vi "LVFinal.vi"() -> ()   [LabVIEW 2016]
panel:
  out "Ball Color":string[](array[string])
  out "Ball Y":dbl[](array[numeric])
  out "Ball X":dbl[](array[numeric])
  in  "Send Button":bool
  in  "DAC2":dbl
  in  "DAC1":dbl
  out "Angle":dbl
  out "Velocity":dbl
  out "Y":dbl
  out "X":dbl
  in  "stop":bool
  in  "Display History":bool
  out "2D Picture":picture
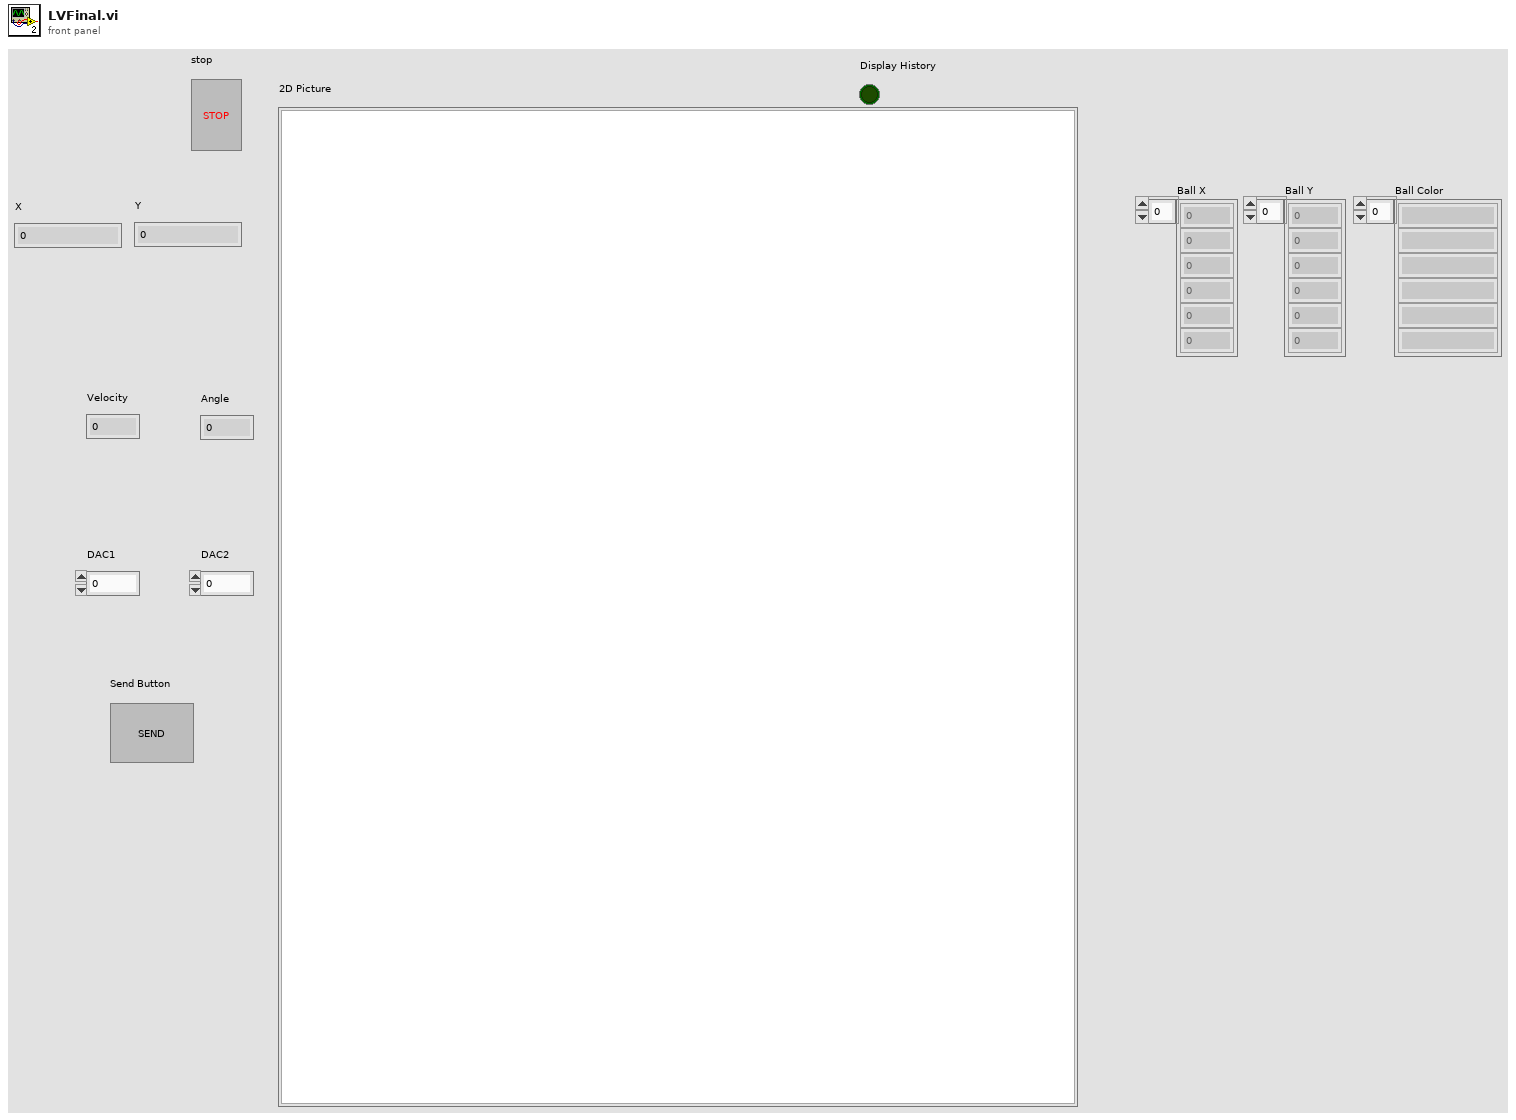
[diagram p1: front panel]
types:
  T1 = cluster{"Width":u16, "Style":enum32{"Solid", "Dash", "Dot", "DashDot", "DashDotDot"}}
  T2 = enum16{"Standard", "Buffered", "CRLF", "Immediate"}
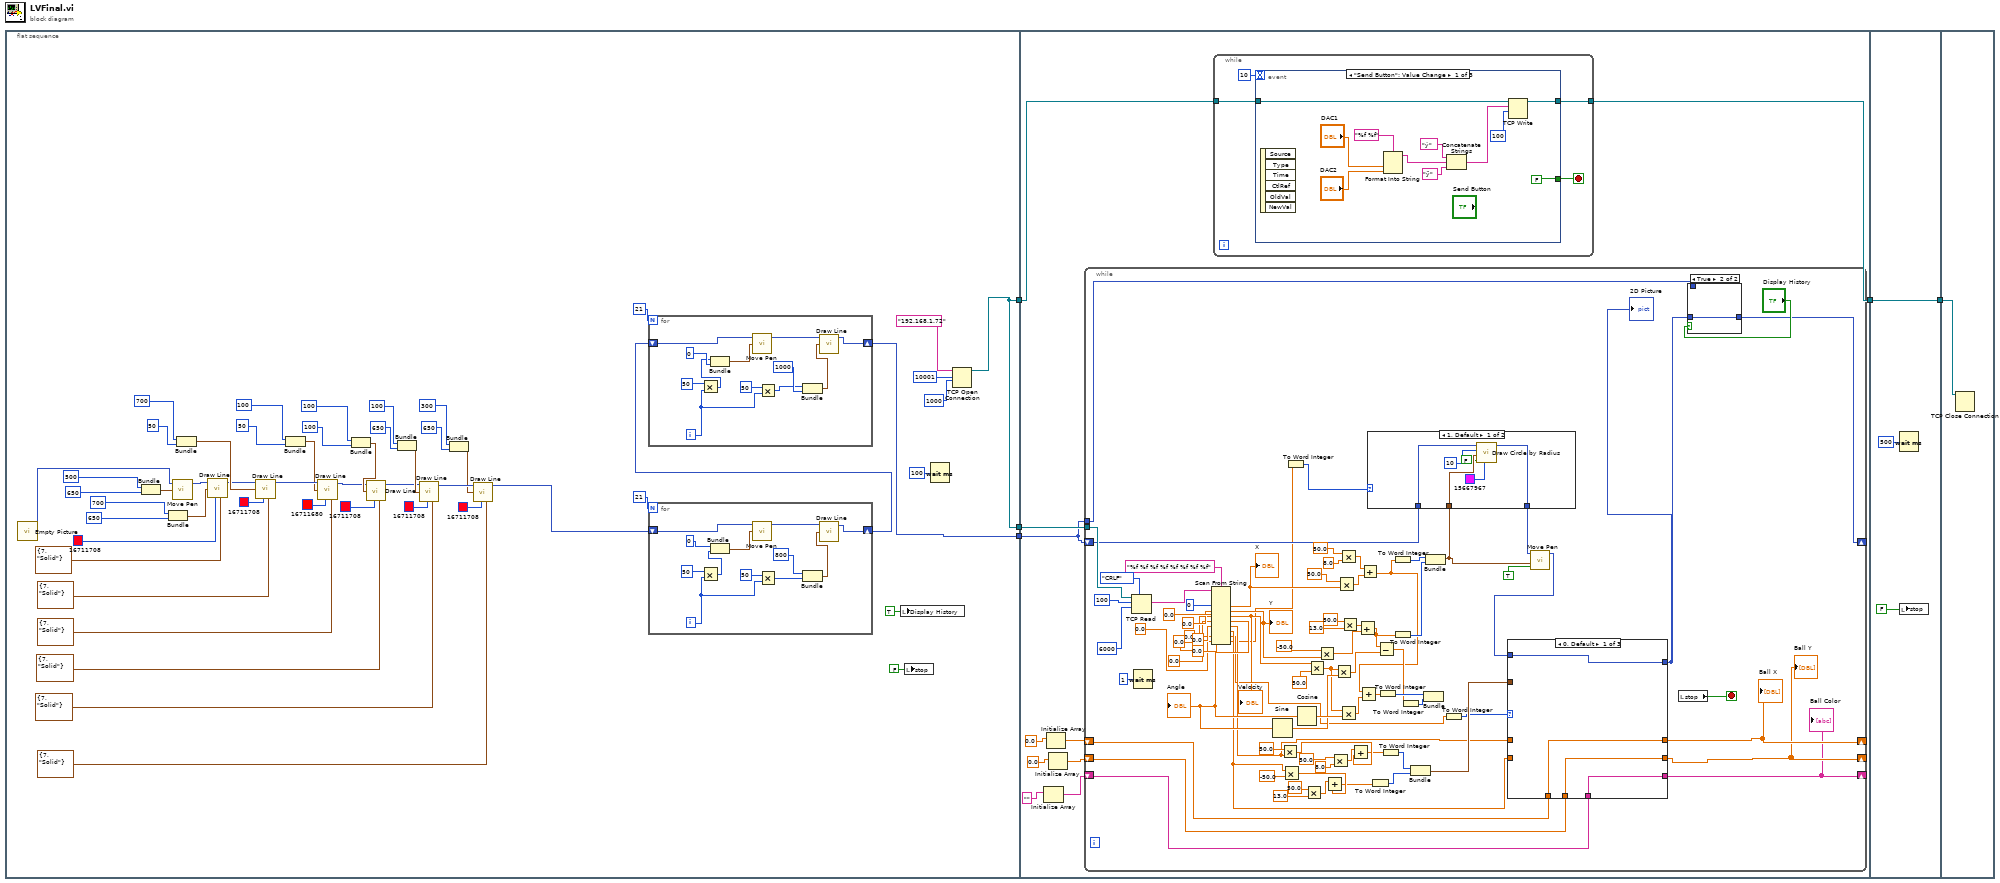
[diagram p0: block diagram]
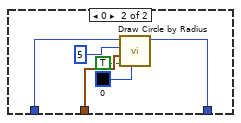
[diagram p2: hidden frame]
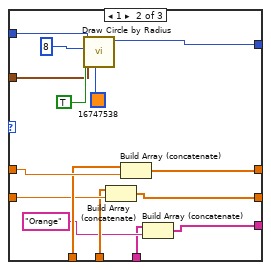
[diagram p3: hidden frame]
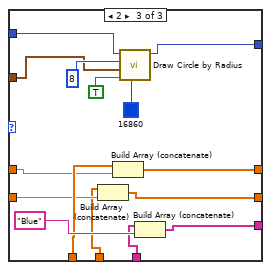
[diagram p4: hidden frame]
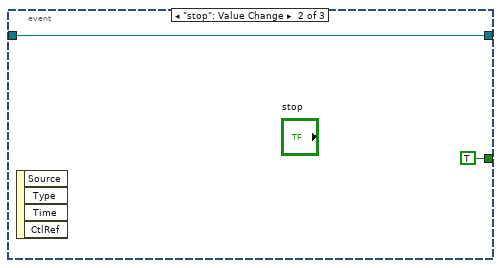
[diagram p6: hidden frame]
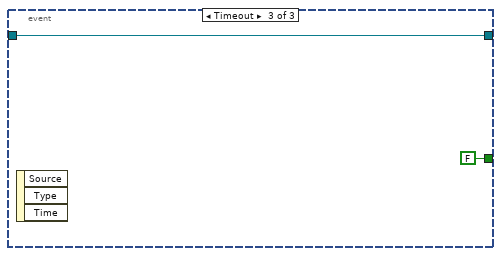
[diagram p7: hidden frame]
diagram:
  n1 = flat-sequence {
    tunnel: [w51] -> w5
    tunnel: [w47] -> w2
    tunnel: [w51] -> w1
    tunnel: w5 -> [w91]
    tunnel: [w90] -> w3
    tunnel: w2 -> [w88]
    tunnel: w1 -> [w89]
    tunnel: [w240] -> w4
    tunnel: w3 -> [w240]
    tunnel: w4 -> [w243]
    frame #0 {
      n2 = call "Empty Picture"() -> ("empty picture"=w39:picture)
      n3 = Bundle(500, 650) -> (w46:cluster{i32, i32})  [unwired: 1 in]
      n4 = Bundle(700, 650) -> (w40:cluster{i32, i32})  [unwired: 1 in]
      n5 = call <vilib>:"Move Pen.vi"("new position"=w46, "picture"=w39) -> ("new picture"=w43:picture)  [unwired: 3 in]
      n6 = Bundle(700, 50) -> (w36:cluster{i32, i32})  [unwired: 1 in]
      n7 = call <vilib>:"Draw Line.vi"("picture"=w43, "end point"=w40, "color(black)"=u32 16711708, "pen"=T1 {"Width"=7, "Style"=enum."Solid"}) -> ("new picture"=w31:picture)  [unwired: 5 in]
      n8 = call <vilib>:"Draw Line.vi"("picture"=w31, "end point"=w36, "color(black)"=u32 16711708, "pen"=T1 {"Width"=7, "Style"=enum."Solid"}) -> ("new picture"=w30:picture)  [unwired: 5 in]
      n9 = Bundle(100, 50) -> (w27:cluster{i32, i32})  [unwired: 1 in]
      n10 = call <vilib>:"Draw Line.vi"("picture"=w30, "end point"=w27, "color(black)"=u32 16711680, "pen"=T1 {"Width"=7, "Style"=enum."Solid"}) -> ("new picture"=w21:picture)  [unwired: 5 in]
      n11 = Bundle(100, 100) -> (w22:cluster{i32, i32})  [unwired: 1 in]
      n12 = call <vilib>:"Draw Line.vi"("picture"=w21, "end point"=w22, "color(black)"=u32 16711708, "pen"=T1 {"Width"=7, "Style"=enum."Solid"}) -> ("new picture"=w17:picture)  [unwired: 5 in]
      n13 = Bundle(100, 650) -> (w18:cluster{i32, i32})  [unwired: 1 in]
      n14 = call <vilib>:"Draw Line.vi"("picture"=w17, "end point"=w18, "color(black)"=u32 16711708, "pen"=T1 {"Width"=7, "Style"=enum."Solid"}) -> ("new picture"=w12:picture)  [unwired: 5 in]
      n15 = Bundle(300, 650) -> (w11:cluster{i32, i32})  [unwired: 1 in]
      n16 = call <vilib>:"Draw Line.vi"("picture"=w12, "end point"=w11, "color(black)"=u32 16711708, "pen"=T1 {"Width"=7, "Style"=enum."Solid"}) -> ("new picture"=w6:picture)  [unwired: 5 in]
      n17 = for {
        N: 21 -> [_]
        shift-right: [w70] -> w48
        shift-left: w6 -> [w72]
        i -> [w71]
        n18 = Multiply(x=50, y=w71) -> (x*y=w74:i32)
        n19 = Bundle(0, w74) -> (w73:cluster{i32, i32})  [unwired: 1 in]
        n20 = call <vilib>:"Move Pen.vi"("new position"=w73, "picture"=w72) -> ("new picture"=w81:picture)  [unwired: 3 in]
        n21 = Multiply(x=50, y=w71) -> (x*y=w79:i32)
        n22 = Bundle(800, w79) -> (w77:cluster{i32, i32})  [unwired: 1 in]
        n23 = call <vilib>:"Draw Line.vi"("picture"=w81, "end point"=w77) -> ("new picture"=w70:picture)  [unwired: 7 in]
      }
      n24 = for {
        N: 21 -> [_]
        shift-right: [w62] -> w47
        shift-left: w48 -> [w64]
        i -> [w63]
        n25 = Multiply(x=50, y=w63) -> (x*y=w60:i32)
        n26 = Bundle(w60, 0) -> (w65:cluster{i32, i32})  [unwired: 1 in]
        n27 = call <vilib>:"Move Pen.vi"("new position"=w65, "picture"=w64) -> ("new picture"=w69:picture)  [unwired: 3 in]
        n28 = Multiply(x=50, y=w63) -> (x*y=w58:i32)
        n29 = Bundle(w58, 1000) -> (w67:cluster{i32, i32})  [unwired: 1 in]
        n30 = call <vilib>:"Draw Line.vi"("picture"=w69, "end point"=w67) -> ("new picture"=w62:picture)  [unwired: 7 in]
      }
      n31 = local write "Display History"(TRUE ("Display History")) -> ()
      n32 = local write "stop"(FALSE ("stop")) -> ()
      n33 = Wait (ms)(milliseconds to wait=u32 100) -> ()  [unwired: 1 out]
      n34 = TCP Open Connection(address="192.168.1.72", remote port or service name=u16 10001, timeout ms (60000)=1000) -> (connection ID=w51:refnum<k5>)  [unwired: 2 in, 1 out]
    }
    frame #1 {
      n35 = Initialize Array("") -> (w83:string[])  [unwired: 1 in]
      n36 = Initialize Array(0.0 ("element")) -> (w87:dbl[])  [unwired: 1 in]
      n37 = Initialize Array(0.0 ("element")) -> (w84:dbl[])  [unwired: 1 in]
      n38 = while {
        shift-right: [w159] -> _
        shift-left: w88 -> [w97]
        tunnel: w89 -> [w158]
        tunnel: w88 -> [w157]
        shift-right: [w106] -> _
        shift-left: w84 -> [w107]
        shift-right: [w108] -> _
        shift-left: w87 -> [w109]
        shift-right: [w104] -> _
        shift-left: w83 -> [w105]
        stop <- w172 stop-if-true
        n39 = TCP Read(connection ID=w158, bytes to read=100, 7:T2."CRLF" ("mode (standard)"), 9:6000 ("timeout ms (25000)")) -> (data out=w167:string)  [unwired: 1 in, 2 out]
        n40 = Wait (ms)(milliseconds to wait=u32 1) -> ()  [unwired: 1 out]
        n41 = Scan From String(format string="%f %f %f %f %f %f %f %f", input string=w167, initial scan location=u32 0, default 1=0.0 ("default value 1"), default 2=0.0 ("default value 2"), default 3=0.0 ("default value 3"), default 4=0.0 ("default value 4"), default 5=0.0 ("default value 5"), default 6=0.0 ("default value 6"), default 7=0.0 ("default value 7"), default 8=0.0 ("default value 8")) -> (output 1=w141:dbl, output 2=w136:dbl, output 3=w99:dbl, output 4=w149:dbl, output 5=w103:dbl, output 6=w102:dbl, output 7=w100:dbl, output 8=w93:dbl)  [unwired: 1 in, 3 out]
        "X" <- w141
        "Y" <- w136
        "Velocity" <- w99
        "Angle" <- w149
        n42 = Sine(x=w149) -> (sin(x)=w148:dbl)
        n43 = Multiply(x=50.0, y=w103) -> (x*y=w118:dbl)
        n44 = Multiply(x=w102, y=-50.0) -> (x*y=w122:dbl)
        n45 = To Word Integer(number=w93) -> (16bit integer=w92:i16)
        n46 = Cosine(x=w149) -> (cos(x)=w150:dbl)
        n47 = Multiply(x=50.0, y=13.0) -> (x*y=w123:dbl)
        n48 = Multiply(x=w99, y=50.0 ("x")) -> (x*y=w129:dbl)
        n49 = Multiply(x=-50.0, y=w136) -> (x*y=w131:dbl)
        n50 = Add(x=w123, y=w122) -> (x+y=w111:dbl)
        n51 = Multiply(x=50.0, y=8.0) -> (x*y=w119:dbl)
        n52 = Multiply(x=w129, y=w148) -> (x*y=w145:dbl)
        n53 = Multiply(x=50.0, y=w141) -> (x*y=w140:dbl)
        n54 = Multiply(x=50.0, y=8.0) -> (x*y=w137:dbl)
        n55 = Multiply(x=w129, y=w150) -> (x*y=w147:dbl)
        n56 = Multiply(x=50.0, y=13.0) -> (x*y=w133:dbl)
        n57 = Add(x=w119, y=w118) -> (x+y=w110:dbl)
        n58 = Add(x=w133, y=w131) -> (x+y=w130:dbl)
        n59 = Add(x=w137, y=w140) -> (x+y=w132:dbl)
        n60 = Add(x=w132, y=w147) -> (x+y=w146:dbl)
        n61 = To Word Integer(number=w111) -> (16bit integer=w116:i16)
        n62 = Subtract(x=w130, y=w145) -> (x-y=w144:dbl)
        n63 = To Word Integer(number=w146) -> (16bit integer=w154:i16)
        n64 = To Word Integer(number=w110) -> (16bit integer=w117:i16)
        n65 = To Word Integer(number=w130) -> (16bit integer=w152:i16)
        n66 = To Word Integer(number=w132) -> (16bit integer=w156:i16)
        n67 = To Word Integer(number=w144) -> (16bit integer=w151:i16)
        n68 = Bundle(w117, w116) -> (w115:cluster{i16, i16})  [unwired: 1 in]
        n69 = Bundle(w154, w151) -> ()  [unwired: 1 in, 1 out]
        n70 = Bundle(w156, w152) -> (w95:cluster{i16, i16})  [unwired: 1 in]
        n71 = case shown="1, Default" w92 {
          tunnel: w97 -> [w177 w183]
          tunnel: [w176 w184] -> w96
          tunnel: w95 -> [w174 w181]
          frame 1, Default {
            n72 = call <vilib>:"Draw Circle by Radius.vi"("color(black)"=u32 15667967, "fill?(F)"=FALSE, "pixel center"=w174, "radius"=i16 10, "picture"=w177) -> ("new picture"=w176:picture)  [unwired: 6 in]
          }
          frame 0 {
            n73 = call <vilib>:"Draw Circle by Radius.vi"("color(black)"=u32 0, "fill?(F)"=TRUE, "pixel center"=w181, "radius"=i16 5, "picture"=w183) -> ("new picture"=w184:picture)  [unwired: 6 in]
          }
        }
        n74 = To Word Integer(number=w100) -> (16bit integer=w112:i16)
        n75 = call <vilib>:"Move Pen.vi"("absolute coordinates?(T)"=TRUE, "new position"=w95, "picture"=w96) -> ("new picture"=w98:picture)  [unwired: 2 in]
        n76 = case shown="0, Default" w112 {
          tunnel: w98 -> [w188 w203 w215]
          tunnel: [w188 w202 w214] -> w128
          tunnel: w115 -> [_ w199 w213]
          tunnel: w102 -> [_ w194 w206]
          tunnel: [w187 w192 w210] -> w106
          tunnel: [w186 w195 w209] -> w108
          tunnel: w103 -> [_ w197 w207]
          tunnel: [w185 w189 w211] -> w104
          tunnel: w109 -> [w186 w196 w208]
          tunnel: w107 -> [w187 w193 w205]
          tunnel: w105 -> [w185 w190 w204]
          frame 0, Default {
          }
          frame 1 {
            n77 = call <vilib>:"Draw Circle by Radius.vi"("color(black)"=u32 16747538, "fill?(F)"=TRUE, "pixel center"=w199, "radius"=i16 8, "picture"=w203) -> ("new picture"=w202:picture)  [unwired: 6 in]
            n78 = Build Array (concatenate)(w193, w194) -> (w192:dbl[])
            n79 = Build Array (concatenate)(w196, w197) -> (w195:dbl[])
            n80 = Build Array (concatenate)(w190, "Orange") -> (w189:string[])
          }
          frame 2 {
            n81 = Build Array (concatenate)(w205, w206) -> (w210:dbl[])
            n82 = Build Array (concatenate)(w208, w207) -> (w209:dbl[])
            n83 = call <vilib>:"Draw Circle by Radius.vi"("color(black)"=u32 16860, "fill?(F)"=TRUE, "pixel center"=w213, "radius"=i16 8, "picture"=w215) -> ("new picture"=w214:picture)  [unwired: 6 in]
            n84 = Build Array (concatenate)(w204, "Blue") -> (w211:string[])
          }
        }
        "2D Picture" <- w128
        "Ball X" <- w108
        "Ball Y" <- w106
        "Ball Color" <- w104
        n85 = local read "stop"() -> (w172:bool)
        n86 = case shown="True" "Display History" {
          tunnel: w128 -> [_ w220]
          tunnel: [w219 w220] -> w159
          tunnel: w157 -> [w219 _]
          frame False {
          }
          frame True {
          }
        }
      }
      n87 = while {
        tunnel: w91 -> [w223]
        tunnel: [w222] -> w90
        stop <- w224 stop-if-true
        n88 = event shown="[0] \"Send Button\": Value Change" {
          selector: _ -> [_ _ _]
          dyn-events: _ -> [_ _ _]
          timeout: 10 -> [_ _ _]
          tunnel: [FALSE TRUE FALSE] -> w224
          tunnel: w223 -> [w226 w236 w239]
          tunnel: [w225 w236 w239] -> w222
          event "Send Button": Value Change {
            n89 = event-data() -> ()  [unwired: 1 in, 6 out]
            n90 = Format Into String(format string="%f %f", "DAC1", "DAC2") -> (resulting string=w233:string)  [unwired: 2 in, 1 out]
            n91 = Concatenate Strings("ý" ("string"), w233, "ÿ" ("string")) -> (w228:string)
            n92 = TCP Write(connection ID=w226, data in=w228, 9:100 ("timeout ms (25000)")) -> (connection ID out=w225:refnum<k5>)  [unwired: 1 in, 2 out]
          }
          event "stop": Value Change {
            n93 = event-data() -> ()  [unwired: 1 in, 4 out]
          }
          event Timeout {
            n94 = event-data() -> ()  [unwired: 1 in, 3 out]
          }
        }
      }
    }
    frame #2 {
      n95 = Wait (ms)(milliseconds to wait=u32 500) -> ()  [unwired: 1 out]
      n96 = local write "stop"(FALSE) -> ()
    }
    frame #3 {
      n97 = TCP Close Connection(connection ID=w243) -> ()  [unwired: 2 in, 2 out]
    }
  }
